vi "state Read.vi"(4 "error in (no error)":errorcluster, 6 "Container State":T4, 7 "Display State In":T2) -> (0 "error out":errorcluster, 2 "Value":cluster{"connect":bool, "Y_State":T1, "Y":dbl}, 3 "Display State Out":T2)   [LabVIEW 2019, in "Heating.lvlib" / "YQ1.xctl"]
uses:
  YQ1.xctl
  <vilib>/_xctls/Container State.ctl
  State.ctl
  Y_state.ctl
  Y_controlState.ctl
  <vilib>/_xctls/XControlSupport.lvlib
  Heating.lvlib
panel:
  # "Replace the Value Indicator below with an Indicator of desired type.\nDo not remove this Indicator or the others from the connector pane. \nDo not change the connector pane pattern.\nThe Value Indicator should always be the second terminal from top on the output side in the connector pane."
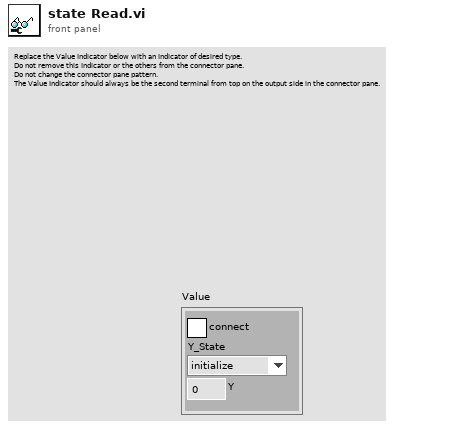
[diagram p1: front panel]
types:
  T1 = typedef "Heating.lvlib/Y_state.ctl" = enum8{"initialize", "alarm", "min", "stop", "hand", "auto", "max"}
  T2 = typedef "Heating.lvlib/YQ1.xctl/State.ctl" = cluster{"Y_State":cluster{"connect":bool, "Y_State":T1, "Y":dbl}, "Write":bool, "button state":T3, "reset_timer":bool, "load_timer":bool, "end_timer":bool}
  T3 = typedef "Heating.lvlib/YQ1.xctl/Y_controlState.ctl" = enum16{"init", "not connect", "alarm", "min", "stop", "hand", "value change", "auto", "max"}
  T4 = typedef "XControlSupport.lvlib/Container State.ctl" = cluster{"Indicator?":bool, "Run Mode?":bool, " Refnum":refnum<vi>}
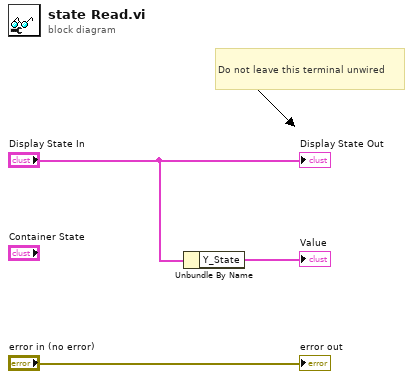
[diagram p0: block diagram]
diagram:
  # "Do not leave this terminal unwired"
  n1 = Unbundle By Name("Display State In") -> ("Y_State"=→"Value":cluster{"connect":bool, "Y_State":T1, "Y":dbl})
  "error out" <- "error in (no error)"
  "Display State Out" <- "Display State In"
